vi "Read_String_From_Excel.vi"(2 "error in (no error)":errorcluster, 3 "Selected Cell":string="A1", 4 "Work Sheet":i32=1, 5 "Excel File Path":path) -> (0 "error out":errorcluster, 1 "Data from Cell":string)   [LabVIEW 2014]
doc: "This example program demonstrates how to read a value from a particular cell in an Excel spreadsheet. Specify the path to an excel file, the worksheet number, and the cell to read and run the VI. The data in the specified file will appear on the front panel."
panel:
  # "Select Help»Show Context Help and move the cursor over the VI icon to display help for this VI"
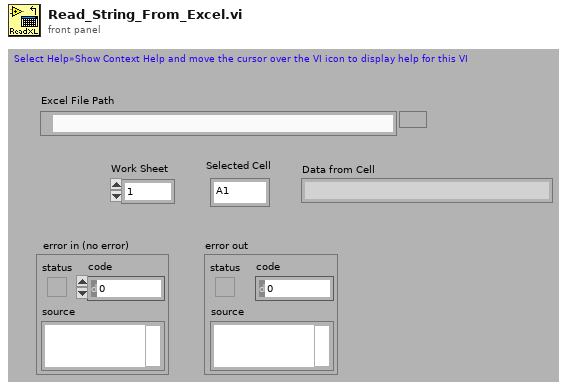
[diagram p1: front panel]
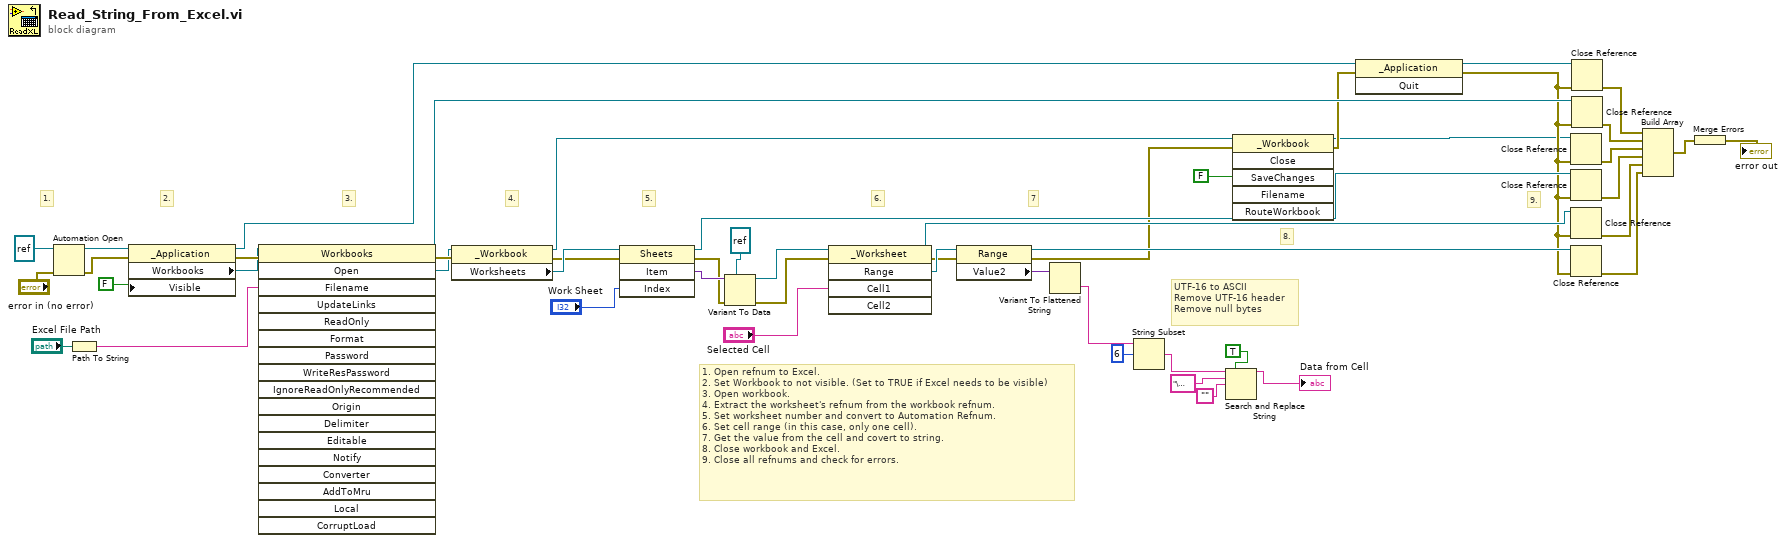
[diagram p0: block diagram]
diagram:
  # "UTF-16 to ASCII\nRemove UTF-16 header\nRemove null bytes"
  # "1. Open refnum to Excel.\n2. Set Workbook to not visible. (Set to TRUE if Excel needs to be visible)\n3. Open workbook.\n4. Extract the worksheet's refnum from the workbook refnum.\n5. Set worksheet number and convert to Automation Refnum.\n6. Set cell range (in this case, only one cell).\n7. Get the value from the cell and covert to string.\n8. Close workbook and Excel.\n9. Close all refnums and check for errors."
  # "9."
  # "8."
  # "7"
  # "6."
  # "5."
  # "4."
  # "3."
  # "2."
  # "1."
  n1 = Automation Open(error in (no error)="error in (no error)", Automation Refnum=refnum<k7> refnum ("Excel._Application")) -> (Automation Refnum=w48:refnum<k7>, error out=w47:errorcluster)  [unwired: 2 in]
  n2 = Path To String(path="Excel File Path") -> (string=w42:string)
  n3 = property class="_Application"(reference=w48, error in=w47, "Visible"=FALSE) -> (reference out=w13:refnum<k7>, error out=w45:errorcluster, "Workbooks"=w44:refnum<k7>)
  n4 = invoke class="Workbooks" method="Open"(reference=w44, error in=w45, "Filename"=w42) -> (reference out=w28:refnum<k7>, error out=w41:errorcluster, "Open"=w40:refnum<k7>)  [unwired: 15 in, 15 out]
  n5 = property class="_Workbook"(reference=w40, error in=w41) -> (reference out=w16:refnum<k7>, error out=w37:errorcluster, "Worksheets"=w38:refnum<k7>)
  n6 = invoke class="Sheets" method="Item"(reference=w38, error in=w37, "Index"="Work Sheet") -> (reference out=w27:refnum<k7>, error out=w34:errorcluster, "Item"=w35:variant)  [unwired: 1 in, 1 out]
  n7 = Variant To Data(error in=w34, type=refnum<k7> refnum ("Excel._Worksheet"), Variant=w35) -> (data=w33:refnum<k7>, error out=w32:errorcluster)
  n8 = invoke class="_Worksheet" method="Range"(reference=w33, error in=w32, "Cell1"="Selected Cell") -> (reference out=w26:refnum<k7>, error out=w29:errorcluster, "Range"=w30:refnum<k7>)  [unwired: 2 in, 2 out]
  n9 = property class="Range"(reference=w30, error in=w29) -> (reference out=w25:refnum<k7>, error out=w9:errorcluster, "Value2"=w8:variant)
  n10 = Variant To Flattened String(Variant=w8) -> (data string=w7:string)  [unwired: 1 out]
  n11 = String Subset(string=w7, offset (0)=6) -> (substring=w2:string)  [unwired: 1 in]
  n12 = Search and Replace String(replace all?=TRUE, input string=w2, search string="\u0000", replace string="") -> (result string=→"Data from Cell":string)  [unwired: 4 in, 3 out]
  n13 = invoke class="_Workbook" method="Close"(reference=w16, error in=w9, "SaveChanges"=FALSE) -> (reference out=w10:refnum<k7>, error out=w12:errorcluster)  [unwired: 3 in, 4 out]
  n14 = invoke class="_Application" method="Quit"(reference=w13, error in=w12) -> (reference out=w14:refnum<k7>, error out=w11:errorcluster)  [unwired: 1 in, 1 out]
  n15 = Close Reference(reference=w10, error in (no error)=w11) -> (error out=w22:errorcluster)
  n16 = Close Reference(reference=w27, error in (no error)=w11) -> (error out=w21:errorcluster)
  n17 = Close Reference(reference=w26, error in (no error)=w11) -> (error out=w20:errorcluster)
  n18 = Close Reference(reference=w25, error in (no error)=w11) -> (error out=w19:errorcluster)
  n19 = Close Reference(reference=w14, error in (no error)=w11) -> (error out=w24:errorcluster)
  n20 = Close Reference(reference=w28, error in (no error)=w11) -> (error out=w23:errorcluster)
  n21 = Build Array(w24, w23, w22, w21, w20, w19) -> (w18:errorcluster[])
  n22 = Merge Errors(w18) -> (→"error out":errorcluster)
